vi "Read Context.vi"(8 "error in (no error)":errorcluster, 11 "DataError in":refnum<class "DataError.lvclass">) -> (0 "error out":errorcluster, 2 "Context":i32(ring)=1 items=["Formatting"=1, "Display"=2, "PreferredSize"=4, "RowDeletion"=8, "Parsing"=256, "Commit"=512, "InitialValueRestoration"=1024, "LeaveControl"=2048, "CurrentCellChange"=4096, "Scroll"=8192, "ClipboardContent"=16384], 3 "DataError out":refnum<class "DataError.lvclass">)   [LabVIEW 2014, in "DataGrid.lvlib" / "DataError.lvclass"]
uses:
  DataError.lvclass
  DataError.lvclass/DataError.ctl
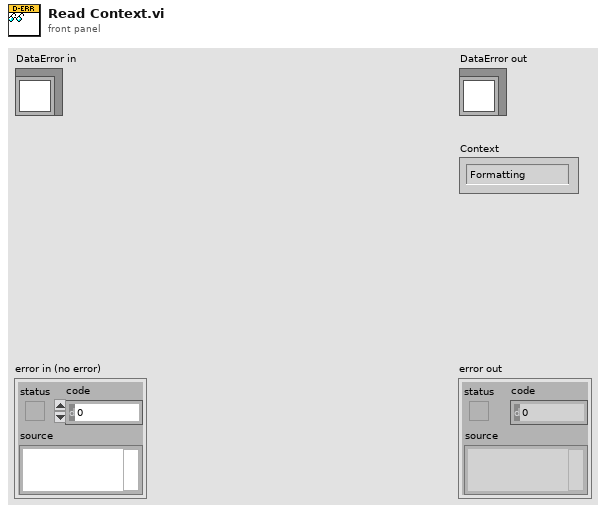
[diagram p1: front panel]
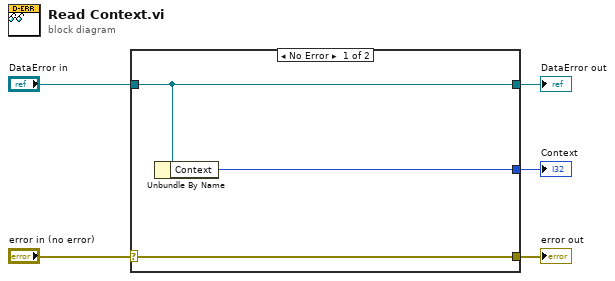
[diagram p0: block diagram]
diagram:
  n1 = case shown="No Error" "error in (no error)" {
    selector: "error in (no error)" -> [w8 w9]
    tunnel: [w8 w9] -> w4
    tunnel: [w7 w10] -> w2
    tunnel: "DataError in" -> [w7 w10]
    tunnel: [w6 _] -> w1
    frame No Error {
      n2 = Unbundle By Name(w7) -> ("Context"=w6:i32)
    }
    frame Error {
    }
  }
  "error out" <- w4
  "DataError out" <- w2
  "Context" <- w1
